vi "Lotto 6 aus 45 – 10 Tipps in Datei.vi"() -> ()   [LabVIEW 2023]
panel:
  out "concatenated string 2":string
  out "concatenated string":string
  out "decimal integer string 2":string
  out "decimal integer string":string
  in  "Dateiname":path
  in  "Start":bool
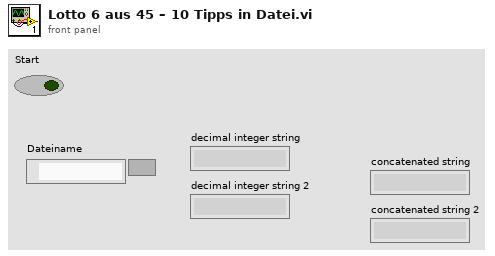
[diagram p1: front panel]
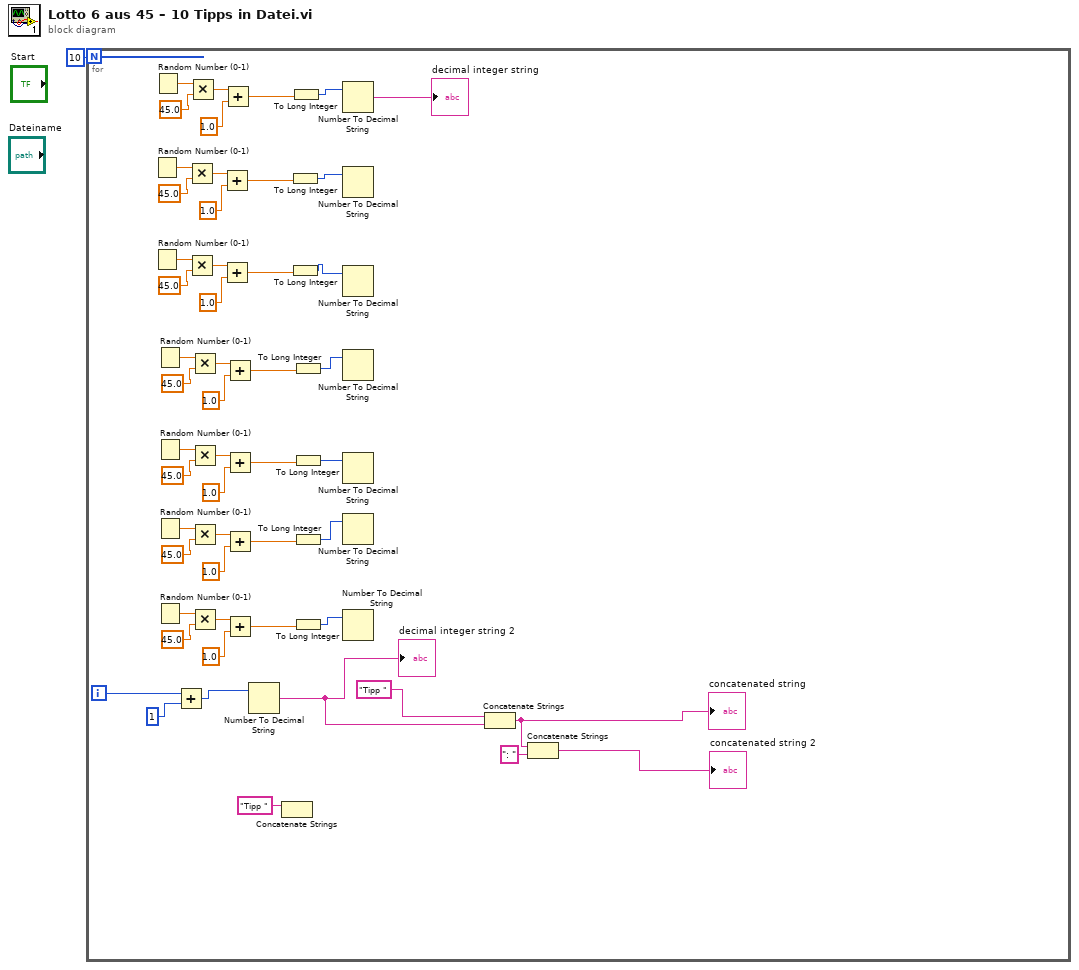
[diagram p0: block diagram]
diagram:
  n1 = for {
    N: 10 -> [_]
    i -> [w11]
    n2 = Random Number (0-1)() -> (number: 0 to 1=w48:dbl)
    n3 = Random Number (0-1)() -> (number: 0 to 1=w33:dbl)
    n4 = Random Number (0-1)() -> (number: 0 to 1=w53:dbl)
    n5 = Random Number (0-1)() -> (number: 0 to 1=w23:dbl)
    n6 = Random Number (0-1)() -> (number: 0 to 1=w38:dbl)
    n7 = Random Number (0-1)() -> (number: 0 to 1=w43:dbl)
    n8 = Random Number (0-1)() -> (number: 0 to 1=w28:dbl)
    n9 = Add(x=w11, y=1) -> (x+y=w9:i32)
    n10 = Multiply(x=w48, y=45.0) -> (x*y=w46:dbl)
    n11 = Multiply(x=w33, y=45.0) -> (x*y=w31:dbl)
    n12 = Multiply(x=w53, y=45.0) -> (x*y=w51:dbl)
    n13 = Multiply(x=w23, y=45.0) -> (x*y=w21:dbl)
    n14 = Multiply(x=w38, y=45.0) -> (x*y=w36:dbl)
    n15 = Multiply(x=w43, y=45.0) -> (x*y=w41:dbl)
    n16 = Multiply(x=w28, y=45.0) -> (x*y=w26:dbl)
    n17 = Add(x=w46, y=1.0) -> (x+y=w44:dbl)
    n18 = Add(x=w31, y=1.0) -> (x+y=w29:dbl)
    n19 = Add(x=w51, y=1.0) -> (x+y=w49:dbl)
    n20 = Add(x=w21, y=1.0) -> (x+y=w19:dbl)
    n21 = Add(x=w36, y=1.0) -> (x+y=w34:dbl)
    n22 = Add(x=w41, y=1.0) -> (x+y=w39:dbl)
    n23 = Add(x=w26, y=1.0) -> (x+y=w24:dbl)
    n24 = Number To Decimal String(number=w9) -> (decimal integer string=w6:string)  [unwired: 1 in]
    "decimal integer string 2" <- w6
    n25 = Concatenate Strings("Tipp " ("string")) -> ()  [unwired: 1 in, 1 out]
    n26 = To Long Integer(number=w44) -> (32bit integer=w17:i32)
    n27 = To Long Integer(number=w29) -> (32bit integer=w16:i32)
    n28 = To Long Integer(number=w49) -> (32bit integer=w18:i32)
    n29 = To Long Integer(number=w19) -> (32bit integer=w15:i32)
    n30 = To Long Integer(number=w34) -> (32bit integer=w14:i32)
    n31 = To Long Integer(number=w39) -> (32bit integer=w13:i32)
    n32 = To Long Integer(number=w24) -> (32bit integer=w12:i32)
    n33 = Number To Decimal String(number=w18) -> (decimal integer string=→"decimal integer string":string)  [unwired: 1 in]
    n34 = Number To Decimal String(number=w17) -> ()  [unwired: 1 in, 1 out]
    n35 = Number To Decimal String(number=w16) -> ()  [unwired: 1 in, 1 out]
    n36 = Number To Decimal String(number=w15) -> ()  [unwired: 1 in, 1 out]
    n37 = Number To Decimal String(number=w14) -> ()  [unwired: 1 in, 1 out]
    n38 = Number To Decimal String(number=w13) -> ()  [unwired: 1 in, 1 out]
    n39 = Number To Decimal String(number=w12) -> ()  [unwired: 1 in, 1 out]
    n40 = Concatenate Strings("Tipp ", w6) -> (w5:string)
    "concatenated string" <- w5
    n41 = Concatenate Strings(w5, ": " ("string")) -> (→"concatenated string 2":string)
  }
